vi "纳清蓝绿藻电极校准.vi"() -> ()   [LabVIEW 2016, in "斯坦道多参数.lvlib"]
uses:
  <vilib>/Utility/miscctls.llb/LVPointTypeDef.ctl
  <vilib>/Utility/miscctls.llb/LVPositionTypeDef.ctl
  <vilib>/Analysis/NI_AALBase.lvlib
panel:
  out "清扫间隔":u16
  out "清扫次数":u16
  in  "清扫模式":u16(ring) items=["自动清扫", "手动清扫", "启动一次清扫"]
  out "滤波设定":sgl
  in  "量程":u16(ring) items=["0-2000000", "0-200000"]
  out "第三点信号值":dbl
  out "第二点信号值":dbl
  out "第一点信号值":dbl
  out "报警信息":string
  out "通讯状态":string
  out "第三点校准值":dbl
  out "标液3":sgl
  out "第二点校准值":dbl
  out "第一点校准值":dbl
  in  "校准停止":bool
  in  "校准启动":bool
  in  "校准模式":u16(ring)=1 items=["两点校准", "单点校准", "三点校准"]
  out "最小值":sgl format="%#.2f"
  out "最大值":sgl format="%#.2f"
  out "波形图表":dbl(graph) caption="历史曲线"
  out "mean":dbl caption="均值" format="%#.2f"
  out "standard deviation":dbl caption="标准差" format="%#.2f"
  out "变异系数":dbl format="%#.6f"
  out "测量值":sgl format="%#.2f"
  out "提示":string
  out "标液2":sgl
  out "标液1":sgl
  out "原始光强数值":u16 caption="信号值"
  out "温度":dbl format="%#.2f"
  # "藻密度电极设定"
  # "℃"
  # "cells/mL"
  # "cells/mL"
  # "请选择校准模式:"
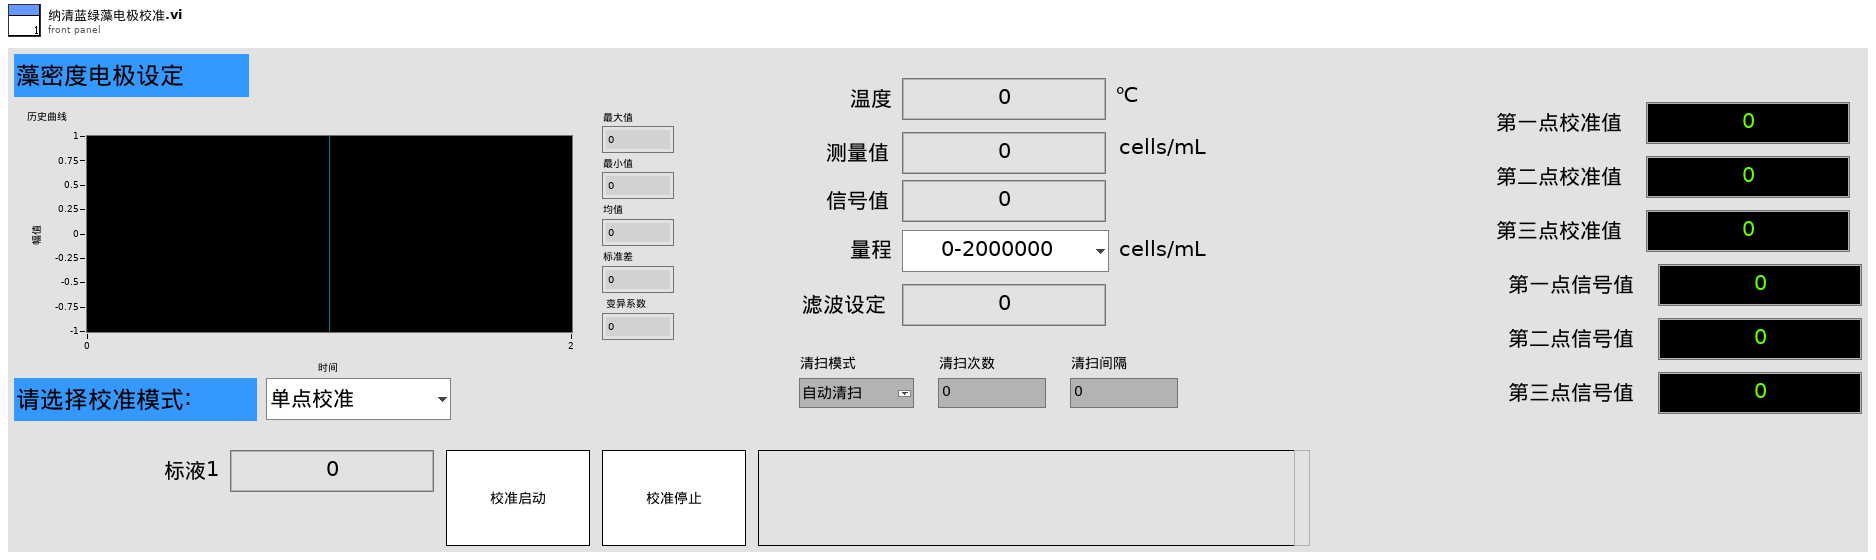
[diagram p1: front panel]
types:
  T1 = typedef "斯坦道多参数.lvlib/通知队列类型.ctl" = enum16{"pH", "DO", "DO2", "Cond", "Turb", "ORP", "叶绿素a", "藻密度", "COD"}
  T2 = typedef "LVPointTypeDef.ctl" = cluster{"Horizontal":i16, "Vertical":i16}
  T3 = cluster{"报警码":u16, "蓝绿藻":sgl, "温度数据":sgl, "原始光强数值":u16, "量程":u16, "平均次数":u16, "清扫模式":u16, "清扫次数":u16, "清扫间隔分钟":u16, "0X000B_NC":string, "产品名称":string, "序列号":string, "硬件版本":string, "软件版本":string, "通讯地址":u16, "波特率":u16, "设备类型":u16, "0X0026_NC":string, "校准量程":u16, "第一点原始光强":u16, "第一点校准数据":sgl, "第二点原始光强":u16, "第二点校准数据":sgl, "第三点原始光强":u16, "第三点校准数据":sgl, "探头校准命令":u16, "温度校准参数":sgl, "温度校准命令":u16}
  T4 = cluster{"pH":u32, "DO":u32, "Cond":u32, "Turb":u32, "叶绿素a":u32, "藻密度":u32, "ORP":u32, "COD":u32}
  T5 = typedef "LVPositionTypeDef.ctl" = cluster{"Left":i32, "Top":i32}
  T6 = enum8{"Enabled", "Disabled", "Disabled and Grayed Out"}
  T7 = cluster{"报警码":u16, "蓝绿藻":sgl, "温度数据":sgl, "原始光强数值":u16, "0X0006_NC":u16, "平均次数":u16, "清扫模式":u16, "清扫次数":u16, "清扫间隔分钟":u16, "0X000B_NC":string, "产品名称":string, "序列号":string, "硬件版本":string, "软件版本":string, "通讯地址":u16, "波特率":u16, "设备类型":u16, "0X0026_NC":string, "0X0030_NC":u16, "第一点原始光强":u16, "第一点校准数据":sgl, "第二点原始光强":u16, "第二点校准数据":sgl, "第三点原始光强":u16, "第三点校准数据":sgl, "探头校准命令":u16, "温度校准参数":sgl, "温度校准命令":u16}
  T8 = cluster{"ph":bool, "DO":bool, "Cond":bool, "Turb":bool, "叶绿素a":bool, "藻密度":bool, "ORP":bool, "COD":bool, "DO2":bool}
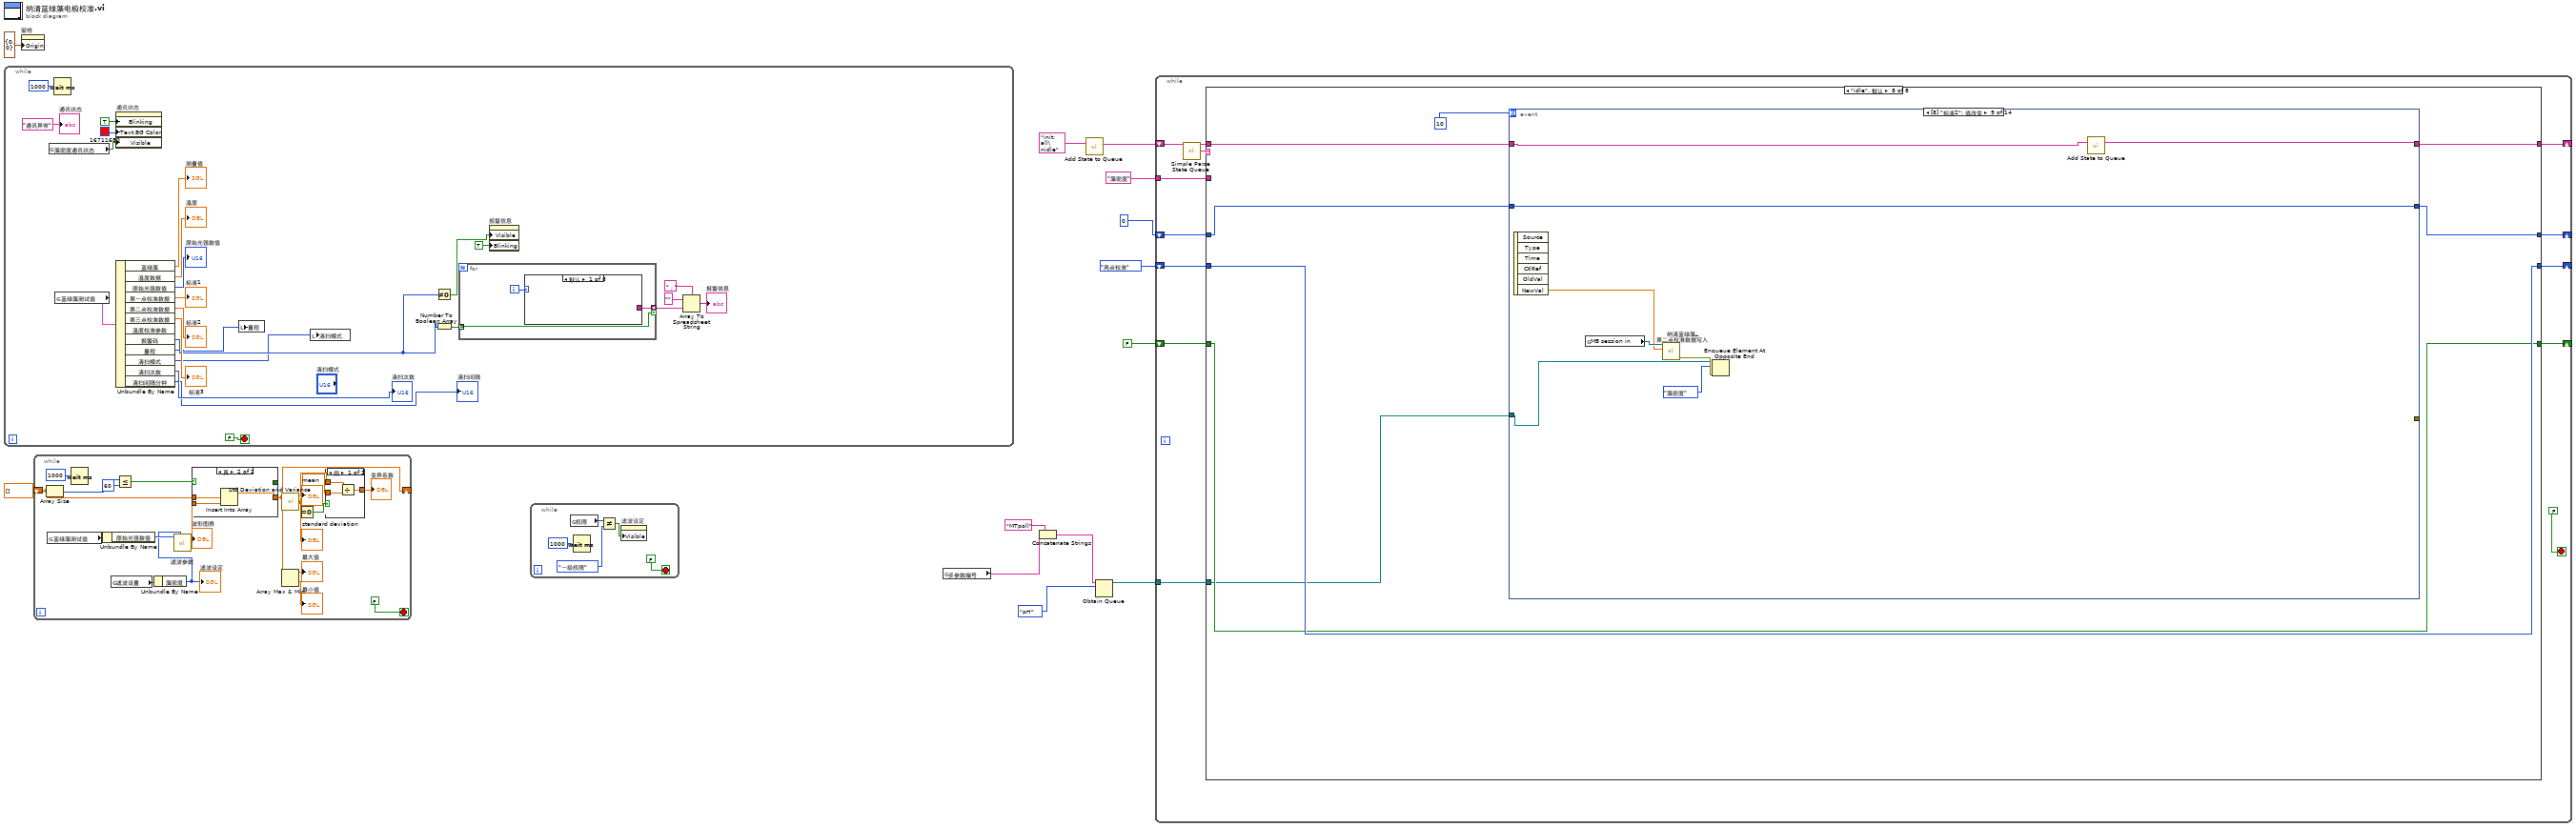
[diagram p0: block diagram]
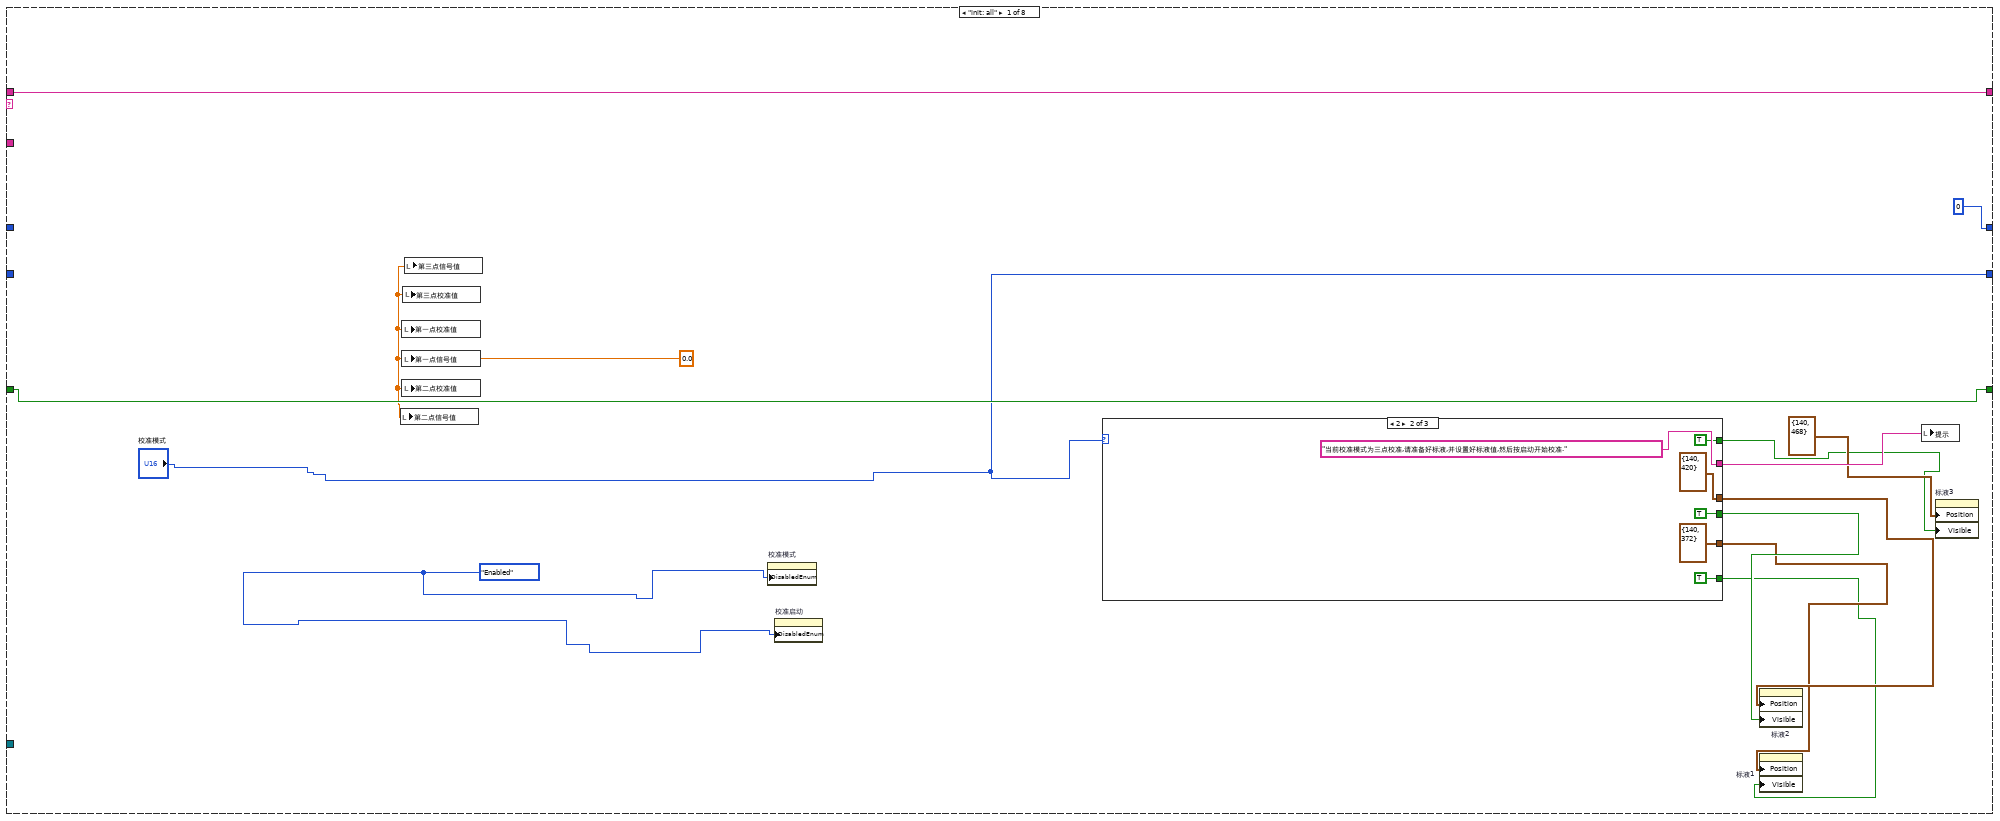
[diagram p2: hidden frame]
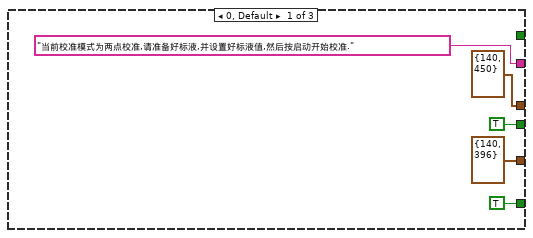
[diagram p3: hidden frame]
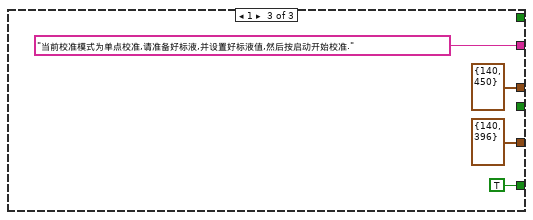
[diagram p4: hidden frame]
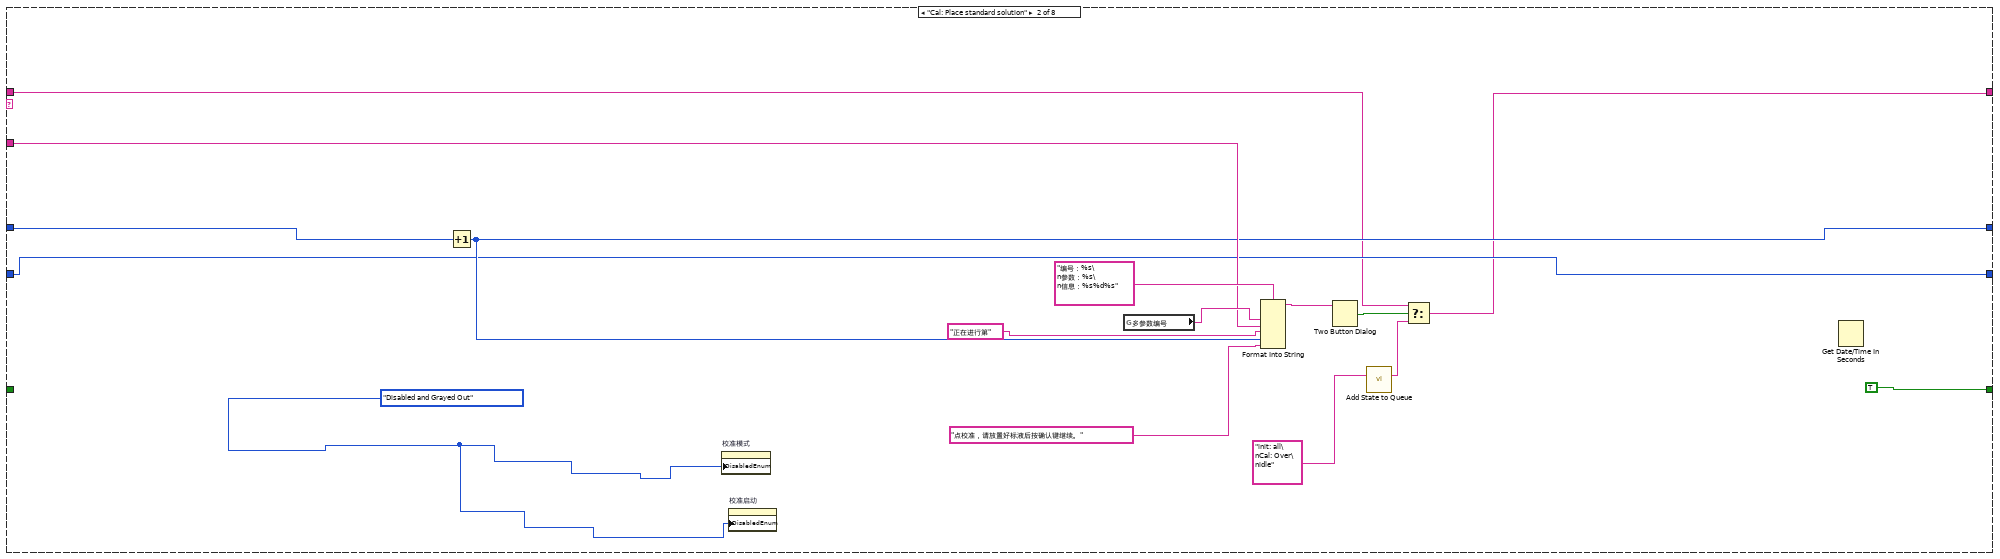
[diagram p5: hidden frame]
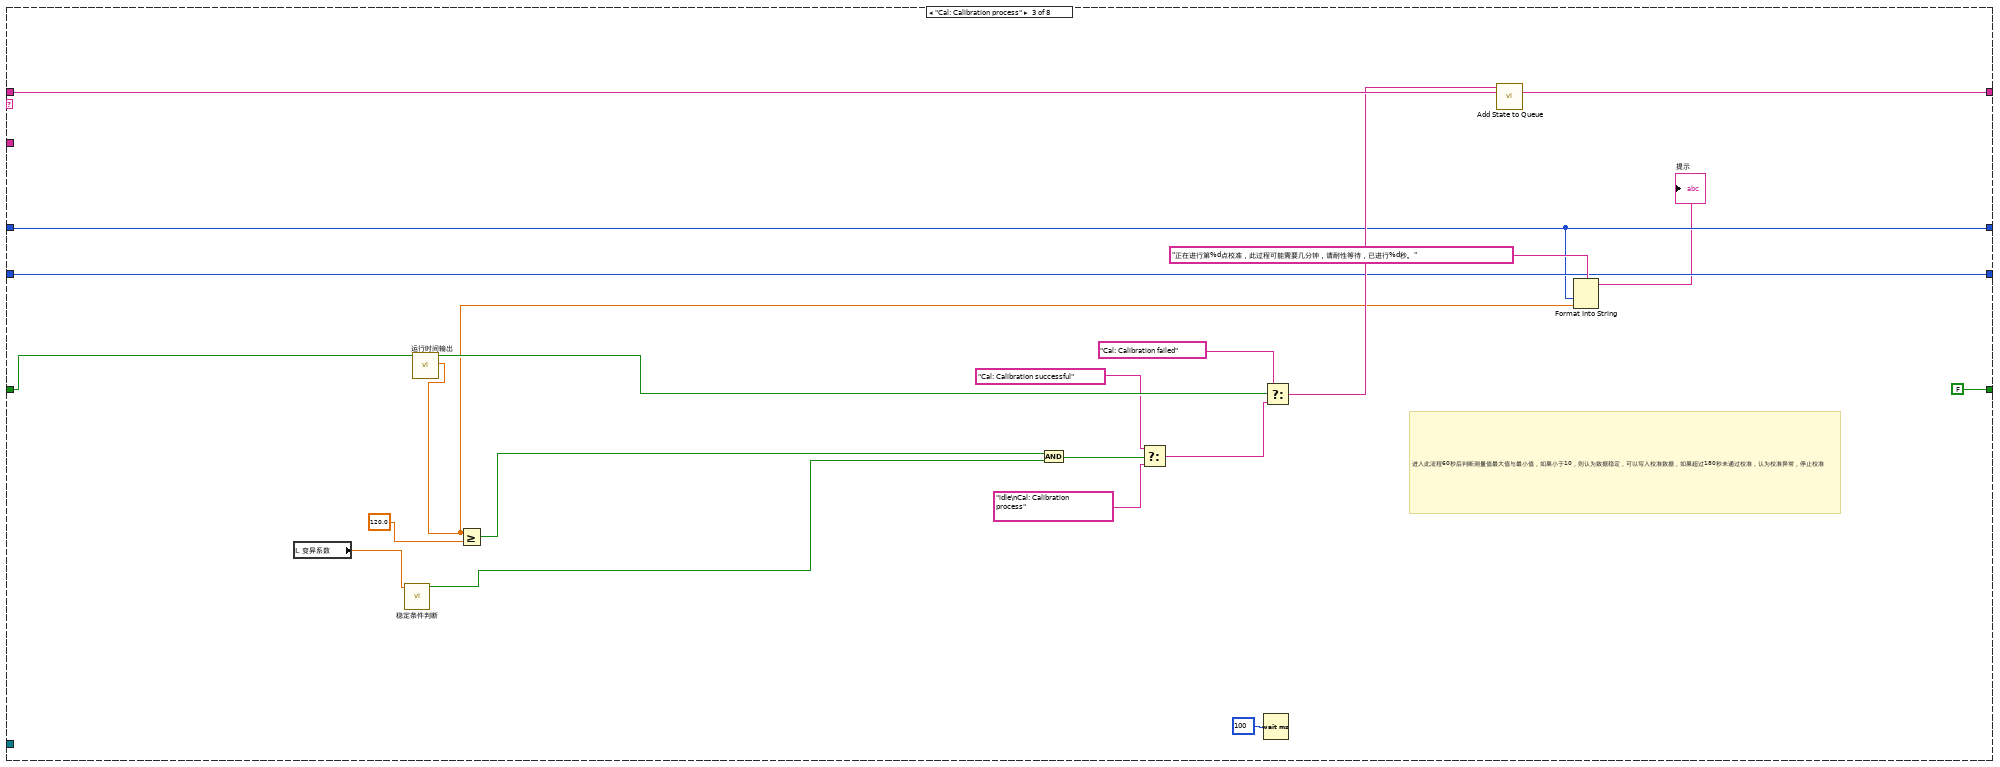
[diagram p6: hidden frame]
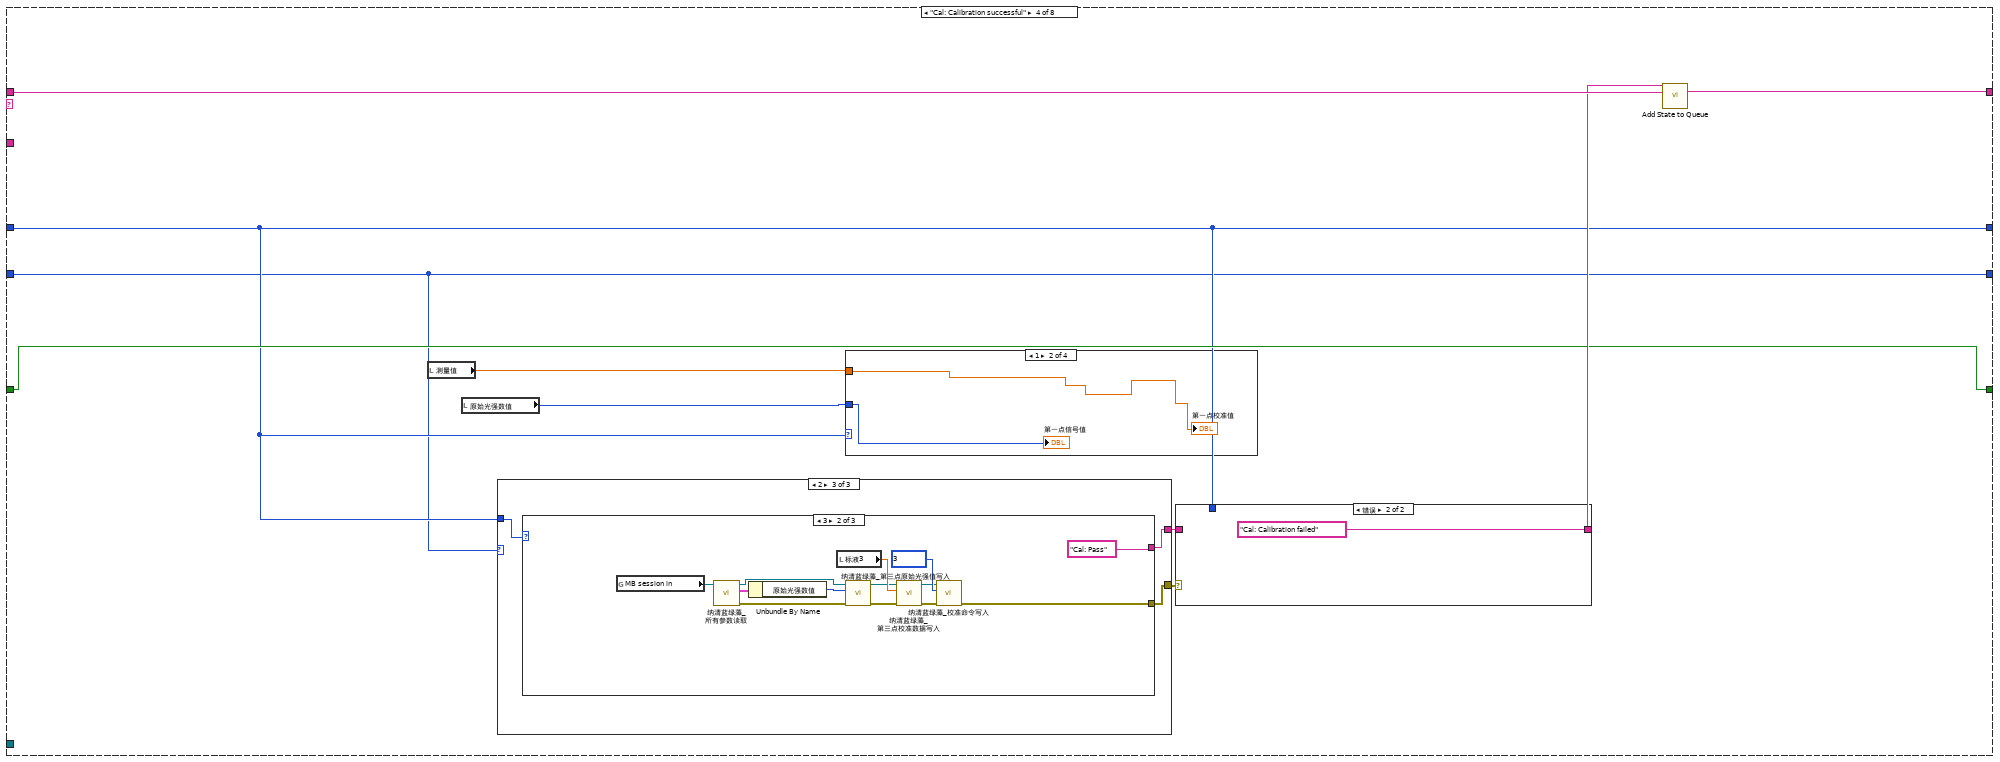
[diagram p7: hidden frame]
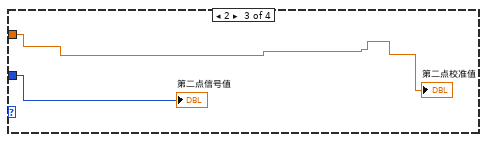
[diagram p9: hidden frame]
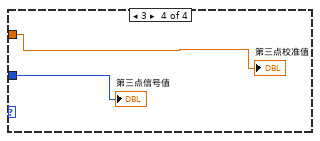
[diagram p10: hidden frame]
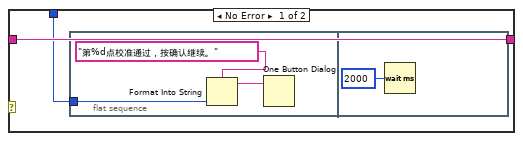
[diagram p11: hidden frame]
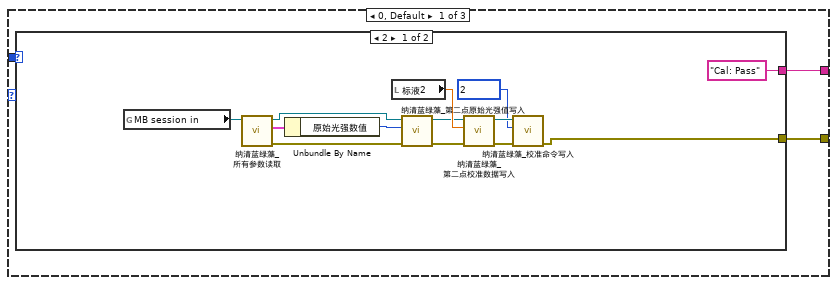
[diagram p12: hidden frame]
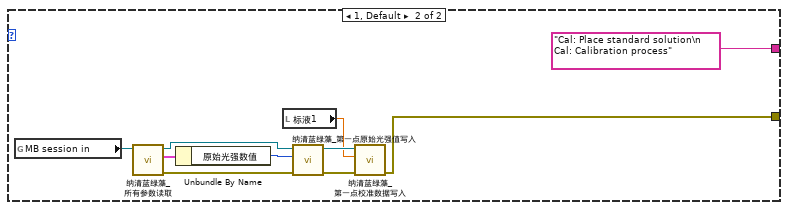
[diagram p13: hidden frame]
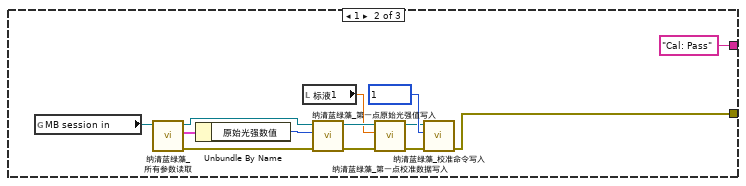
[diagram p14: hidden frame]
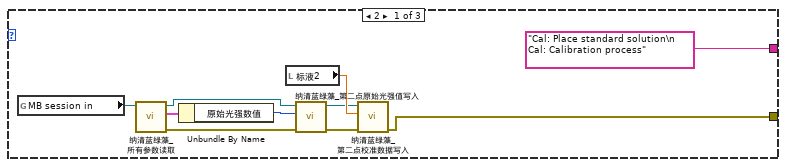
[diagram p15: hidden frame]
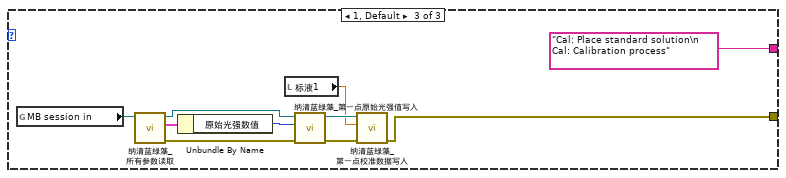
[diagram p16: hidden frame]
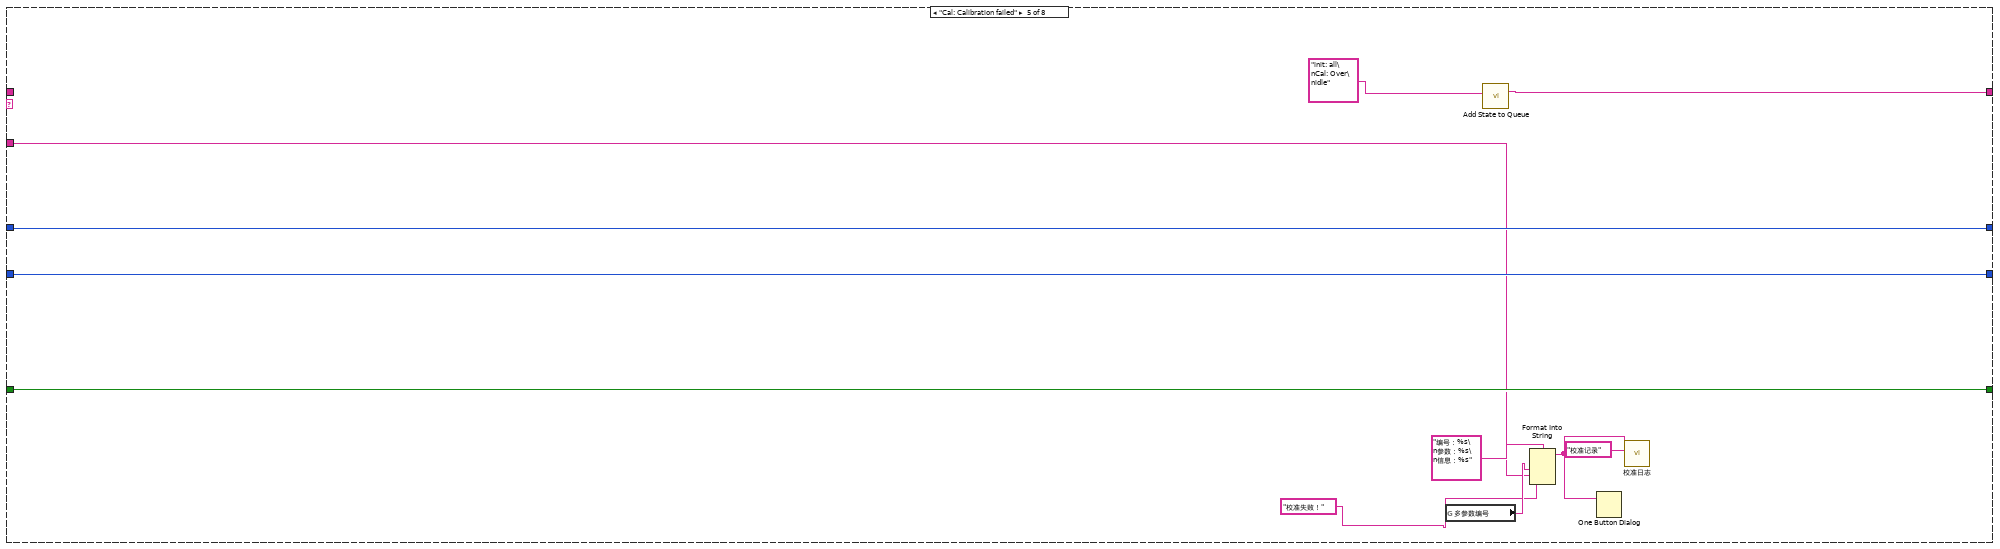
[diagram p17: hidden frame]
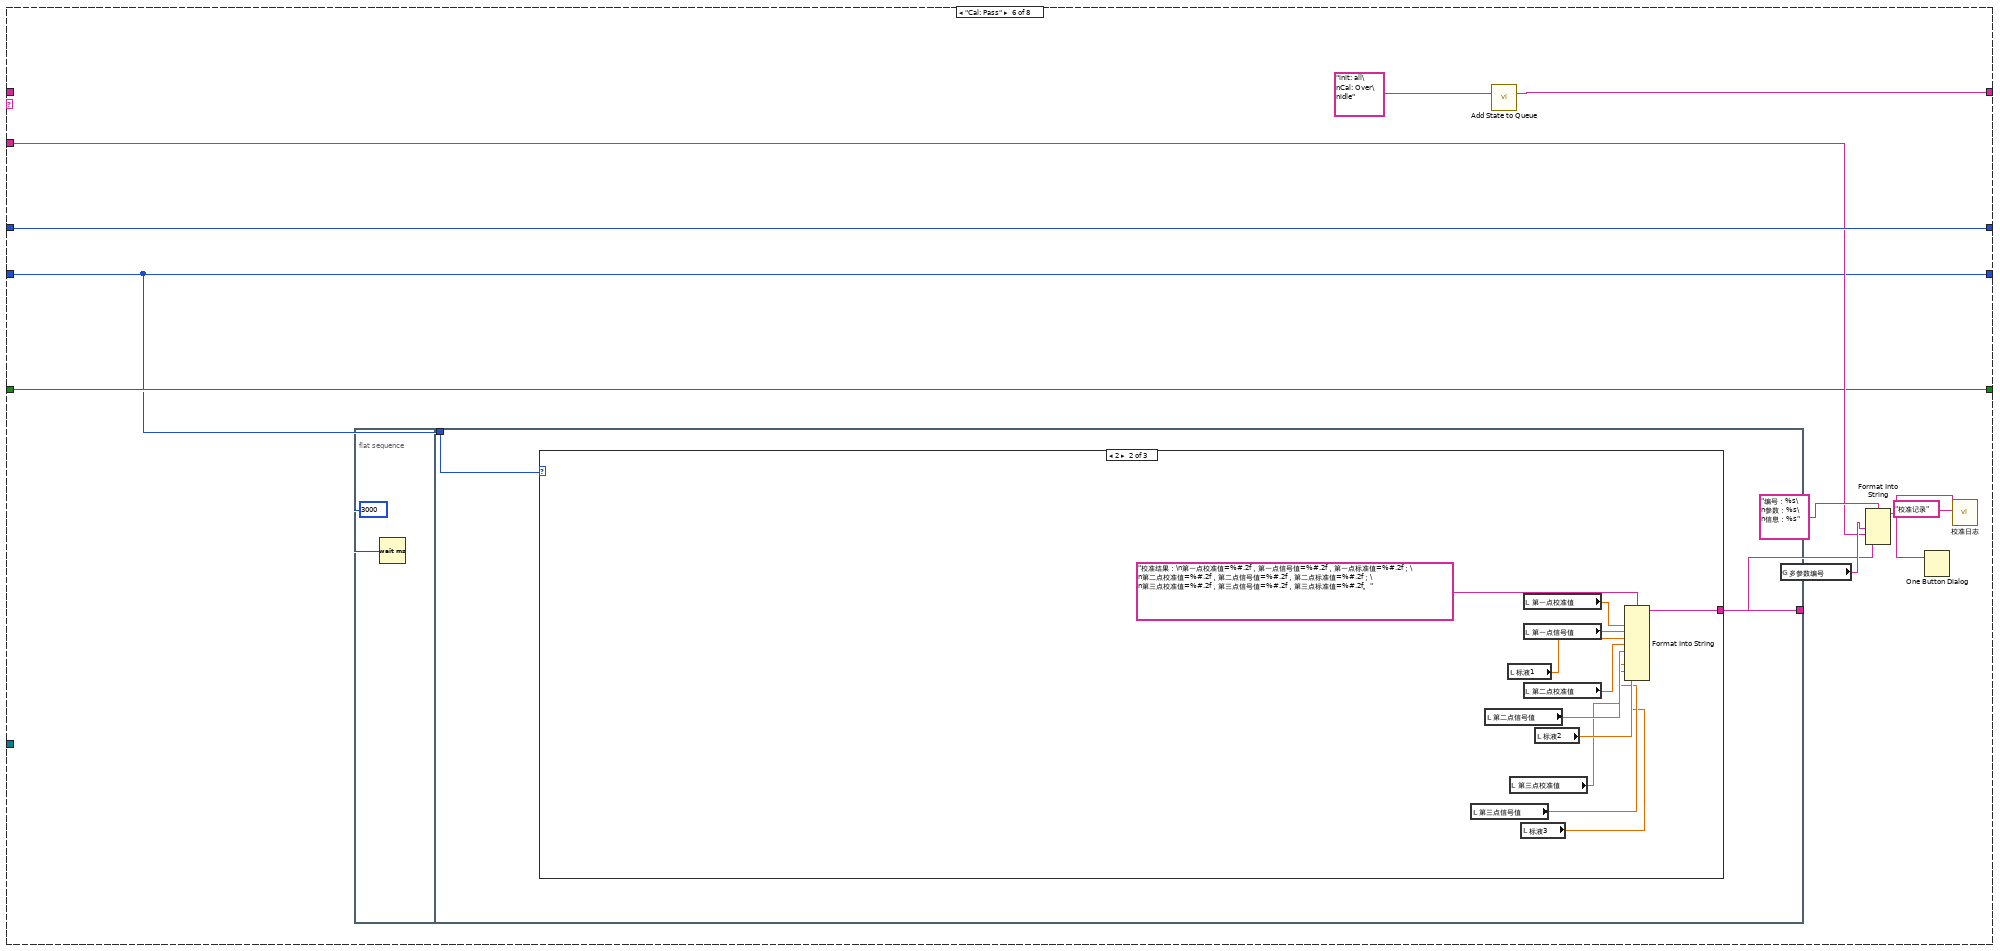
[diagram p18: hidden frame]
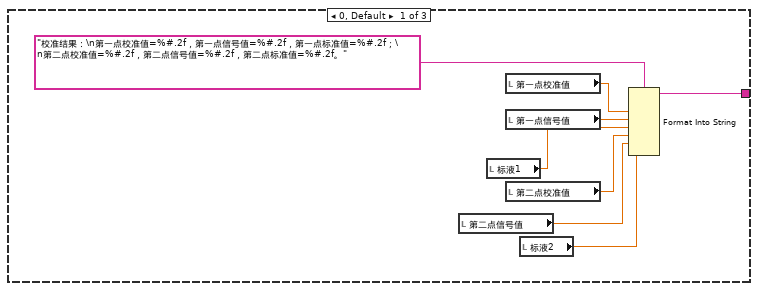
[diagram p19: hidden frame]
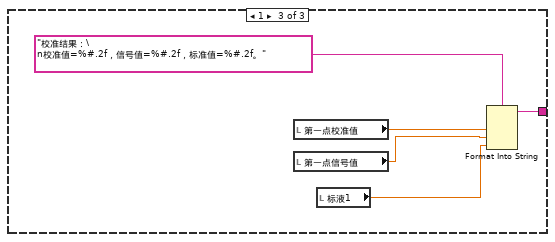
[diagram p20: hidden frame]
diagram:
  n1 = while {
    stop <- FALSE stop-if-true
    n2 = global read "多参数全局变量.vi" "藻密度通讯状态"() -> (w26:bool)
    n3 = Wait (ms)(milliseconds to wait=u32 1000 ("等待时间（毫秒）")) -> ()  [unwired: 1 out]
    n4 = global read "纳清过程全局变量.vi" "蓝绿藻测试值"() -> (w36:T3)
    n5 = property on="通讯状态" class="Str"("Blinking"=TRUE ("闪烁"), "Text.BG Color"=u32 16711680, "Visible"=w26) -> ()  [unwired: 2 in, 2 out]
    n6 = Unbundle By Name(w36) -> ("蓝绿藻"=→"测量值":sgl, "温度数据"=→"温度":sgl, "原始光强数值"=→"原始光强数值":u16, "第一点校准数据"=→"标液1":sgl, "第二点校准数据"=→"标液2":sgl, "第三点校准数据"=→"标液3":sgl, "报警码"=w18:u16, "量程"=w17:u16, "清扫模式"=w14:u16, "清扫次数"=→"清扫次数":u16, "清扫间隔分钟"=→"清扫间隔":u16)  [unwired: 1 out]
    n7 = local write "量程"(w17) -> ()
    n8 = local write "清扫模式"(w14) -> ()
    n9 = Not Equal To 0?(x=w18) -> (x != 0?=w20:bool)
    n10 = Number To Boolean Array(number=w18) -> (Boolean array=w25:bool[])
    n11 = for {
      tunnel: w25 -> [w39] mode=indexing
      tunnel: [w40] -> w24 mode=indexing if=w39
      i -> [w41]
      n12 = case shown="默认" w41 {
        tunnel: [_ "测量值超量程" "温度超量程" "光强信号超范围" "清扫中" "温度传感器故障" "电极故障" "内部电压基准故障"] -> w40
        frame Default {
        }
        frame 0 {
        }
        frame 2 {
        }
        frame 3 {
        }
        frame 4 {
        }
        frame 8 {
        }
        frame 9 {
        }
        frame 10 {
        }
      }
    }
    n13 = property on="报警信息" class="Str"("Visible"=w20, "Blinking"=TRUE ("闪烁")) -> ()  [unwired: 2 in, 2 out]
    n14 = Array To Spreadsheet String(delimiter (Tab)="；" ("分隔符(Tab)"), array=w24, 3:"" ("格式字符串")) -> (spreadsheet string=→"报警信息":string)
    "通讯状态" <- "通讯异常" ("当前串口")
  }
  n15 = property on="窗格" class="Pane"("Origin"=T2 {"Horizontal"=0, "Vertical"=0} ("原点")) -> ()  [unwired: 2 in, 2 out]
  n16 = while {
    shift-right: [w56] -> _
    shift-left: sgl[] [] -> [w62]
    stop <- FALSE stop-if-true
    n17 = Array Size(array=w62) -> (size(s)=w64:i32)
    n18 = global read "纳清过程全局变量.vi" "蓝绿藻测试值"() -> (w53:T3)
    n19 = Wait (ms)(milliseconds to wait=u32 1000 ("等待时间（毫秒）")) -> ()  [unwired: 1 out]
    n20 = Unbundle By Name(w53) -> ("原始光强数值"=w52:u16)
    n21 = global read "断电保存变量.vi" "滤波设置"() -> (w50:T4)
    n22 = Less Or Equal?(x=w64, y=60) -> (x <= y?=w63:bool)
    n23 = Unbundle By Name(w50) -> ("藻密度"=w49:u32)
    "滤波设定" <- w49
    n24 = call "滤波参数.vi"("滤波次数"=w49, "x"=w52) -> ("mode"=w51:dbl)  [unwired: 9 in]
    "波形图表" <- w51
    n25 = case shown="真" w63 {
      tunnel: w62 -> [w75 w78]
      tunnel: w51 -> [w73 w77]
      tunnel: [w71 w76] -> w56
      tunnel: [TRUE _] -> _
      frame False {
        n26 = Replace Array Subset(array=w75, new element=w73) -> (w74:sgl[])  [unwired: 1 in]
        n27 = Rotate 1D Array(1:w74, 2:-1 ("n")) -> (0:w71:sgl[])
      }
      frame True {
        n28 = Insert Into Array(array=w78, new element=w77) -> (w76:sgl[])  [unwired: 1 in]
      }
    }
    n29 = call <vilib>:"Std Deviation and Variance.vi"("X"=w56) -> ("mean"=w60:dbl, "standard deviation"=w59:dbl)  [unwired: 1 in, 1 out]
    "mean" <- w60
    "standard deviation" <- w59
    n30 = Array Max & Min(array=w56) -> (max value=→"最大值":sgl, min value=→"最小值":sgl)  [unwired: 2 out]
    n31 = Equal To 0?(x=w60) -> (x = 0?=w61:bool)
    n32 = case shown="假" w61 {
      tunnel: w59 -> [w69 _]
      tunnel: [w68 _] -> w58
      tunnel: w60 -> [w67 _]
      frame False {
        n33 = Divide(x=w69, y=w67) -> (x/y=w68:dbl)
      }
      frame True {
      }
    }
    "变异系数" <- w58
  }
  n34 = while {
    stop <- FALSE stop-if-true
    n35 = global read "多参数全局变量.vi" "权限"() -> (w82:enum16{"一级权限", "二级权限", "三级权限"})
    n36 = Wait (ms)(milliseconds to wait=u32 1000 ("等待时间（毫秒）")) -> ()  [unwired: 1 out]
    n37 = Not Equal?(x=w82, y=enum16{"一级权限", "二级权限", "三级权限"}."一级权限") -> (x != y?=w79:bool)
    n38 = property on="滤波设定" class="DigNum (严格)"("Visible"=w79) -> ()  [unwired: 2 in, 2 out]
  }
  n39 = global read "多参数全局变量.vi" "多参数编号"() -> (w3:string)
  n40 = Concatenate Strings("MTpoll" ("名称（未命名）"), w3) -> (w4:string)
  n41 = call "Add State to Queue.vi"("State(s) In (\"\")"="init: all\nidle" ("State(s) In (\"\")")) -> ("States Out"=w10:string)  [unwired: 14 in]
  n42 = Obtain Queue(name (unnamed)=w4, element data type=通知队列类型."pH" ("枚举")) -> (queue out=w2:refnum<queue>)  [unwired: 3 in, 2 out]
  n43 = while {
    shift-right: [w92] -> _
    shift-left: w10 -> [w96]
    shift-right: [w89] -> _
    shift-left: 0 -> [w91]
    tunnel: "藻密度" ("State(s) In (\"\")") -> [w90]
    shift-right: [w87] -> _
    shift-left: enum16{"两点校准", "单点校准", "三点校准"}."两点校准" ("校准模式") -> [w88]
    shift-right: [w85] -> _
    shift-left: FALSE -> [w86]
    tunnel: w2 -> [w84]
    stop <- FALSE stop-if-true
    n44 = call "Simple Parse State Queue.vi"("State Queue"=w96) -> ("Remain States"=w93:string, "Next State"=w94:string)  [unwired: 13 in]
    n45 = case shown="\"idle\", 默认" w94 {
      tunnel: w93 -> [w109 w128 w160 w169 _ _ w312 w323]
      tunnel: [w109 w127 w159 w168 w267 w272 w312 w322] -> w92
      tunnel: w91 -> [_ w136 w145 w163 w270 w281 w311 w320]
      tunnel: w90 -> [_ w137 _ _ w261 w277 _ _]
      tunnel: [0 w134 w145 w163 w270 w281 w311 w321] -> w89
      tunnel: w88 -> [_ w133 w146 w162 w269 w273 w310 w319]
      tunnel: ["校准模式" w133 w146 w162 w269 w273 w310 w319] -> w87
      tunnel: w86 -> [w107 _ w148 w164 w268 w276 w309 w317]
      tunnel: [w107 TRUE FALSE w164 w268 w276 w309 w317] -> w85
      tunnel: w84 -> [_ _ _ _ _ _ _ w316]
      frame "init: all" {
        w103 = T6."Enabled" ("禁用")
        w106 = 0.0 ("第一点校准值")
        n46 = local write "第二点信号值"(w106) -> ()
        n47 = local write "第一点校准值"(w106) -> ()
        n48 = local write "第一点信号值"(w106) -> ()
        n49 = local write "第二点校准值"(w106) -> ()
        n50 = local write "第三点校准值"(w106) -> ()
        n51 = local write "第三点信号值"(w106) -> ()
        n52 = property on="校准模式" class="Ring (严格)"("DisabledEnum"=w103) -> ()  [unwired: 2 in, 2 out]
        n53 = property on="校准启动" class="Bool"("DisabledEnum"=w103) -> ()  [unwired: 2 in, 2 out]
        n54 = case shown="2" "校准模式" {
          tunnel: ["当前校准模式为两点校准,请准备好标液,并设置好标液值,然后按启动开始校准." ("提示") "当前校准模式为三点校准,请准备好标液,并设置好标液值,然后按启动开始校准." ("提示") "当前校准模式为单点校准,请准备好标液,并设置好标液值,然后按启动开始校准." ("提示")] -> w105
          tunnel: [TRUE ("可见") TRUE ("可见") _] -> w99
          tunnel: [T5 {"Left"=140, "Top"=396} ("位置") T5 {"Left"=140, "Top"=372} ("位置") T5 {"Left"=140, "Top"=396} ("位置")] -> w98
          tunnel: [T5 {"Left"=140, "Top"=450} ("位置 2") T5 {"Left"=140, "Top"=420} ("位置 2") T5 {"Left"=140, "Top"=450} ("位置 2")] -> w100
          tunnel: [_ TRUE ("可见") _] -> w101
          tunnel: [TRUE ("可见") TRUE ("可见") TRUE ("可见")] -> w97
          frame 0, Default {
          }
          frame 2 {
          }
          frame 1 {
          }
        }
        n55 = property on="标液2" class="DigNum (严格)"("Position"=w100, "Visible"=w99) -> ()  [unwired: 2 in, 2 out]
        n56 = property on="标液1" class="DigNum (严格)"("Position"=w98, "Visible"=w97) -> ()  [unwired: 2 in, 2 out]
        n57 = local write "提示"(w105) -> ()
        n58 = property on="标液3" class="DigNum (严格)"("Position"=T5 {"Left"=140, "Top"=468} ("位置 3"), "Visible"=w101) -> ()  [unwired: 2 in, 2 out]
      }
      frame "Cal: Place standard solution" {
        w126 = T6."Disabled and Grayed Out" ("禁用")
        n59 = Increment(x=w136) -> (x+1=w134:i32)
        n60 = property on="校准模式" class="Ring (严格)"("DisabledEnum"=w126) -> ()  [unwired: 2 in, 2 out]
        n61 = property on="校准启动" class="Bool"("DisabledEnum"=w126) -> ()  [unwired: 2 in, 2 out]
        n62 = global read "多参数全局变量.vi" "多参数编号"() -> (w139:string)
        n63 = Format Into String(format string="编号：%s\n参数：%s\n信息：%s%d%s" ("格式字符串"), w139, w137, "正在进行第" ("消息"), w134, "点校准，请放置好标液后按确认键继续。" ("消息")) -> (resulting string=w131:string)  [unwired: 2 in, 1 out]
        n64 = Two Button Dialog(message=w131) -> (T button?=w130:bool)  [unwired: 2 in]
        n65 = call "Add State to Queue.vi"("State(s) In (\"\")"="init: all\nCal: Over\nidle" ("State(s) In (\"\")")) -> ("States Out"=w129:string)  [unwired: 14 in]
        n66 = Select(t=w128, s=w130, f=w129) -> (s? t:f=w127:string)
        n67 = Get Date/Time In Seconds() -> ()  [unwired: 1 out]
      }
      frame "Cal: Calibration process" {
        # "进入此流程60秒后判断测量值最大值与最小值，如果小于10，则认为数据稳定，可以写入校准数据，如果超过180秒未通过校准，认为校准异常，停止校准"
        n68 = local read "变异系数"() -> (w142:dbl)
        n69 = call "稳定条件判断.vi"("变异系数"=w142) -> ("布尔"=w141:bool)  [unwired: 10 in]
        n70 = call "运行时间输出.vi"("初始化"=w148) -> ("Elapsed Time (s)"=w144:dbl, "Time has Elapsed"=w161:bool)  [unwired: 9 in]
        n71 = Greater Or Equal?(x=w144, y=120.0) -> (x >= y?=w156:bool)
        n72 = And(x=w156, y=w141) -> (x .and. y?=w153:bool)
        n73 = Select(t="Cal: Calibration successful" ("State(s) In (\"\")"), s=w153, f="idle\nCal: Calibration process" ("State(s) In (\"\")")) -> (s? t:f=w152:string)
        n74 = Wait (ms)(milliseconds to wait=u32 100 ("等待时间（毫秒）")) -> ()  [unwired: 1 out]
        n75 = Select(t="Cal: Calibration failed" ("State(s) In (\"\")"), s=w161, f=w152) -> (s? t:f=w151:string)
        n76 = call "Add State to Queue.vi"("State(s) In Front (\"\")"=w151, "State(s) In (\"\")"=w160) -> ("States Out"=w159:string)  [unwired: 13 in]
        n77 = Format Into String(format string="正在进行第%d点校准，此过程可能需要几分钟，请耐性等待，已进行%d秒。" ("格式字符串"), w145, w144) -> (resulting string=→"提示":string)  [unwired: 2 in, 1 out]
      }
      frame "Cal: Calibration successful" {
        n78 = local read "测量值"() -> (w165:sgl)
        n79 = local read "原始光强数值"() -> (w166:u16)
        n80 = case shown="2" w162 {
          tunnel: [w187 w211 w224] -> w171
          tunnel: [w186 "Cal: Pass" ("State(s) In (\"\")") w225] -> w170
          tunnel: w163 -> [w185 _ w226]
          frame 0, Default {
            n81 = case shown="2" w185 {
              tunnel: [w188 w201] -> w187
              tunnel: ["Cal: Pass" ("State(s) In (\"\")") "Cal: Place standard solution\n Cal: Calibration process" ("State(s) In (\"\")")] -> w186
              frame 2 {
                n82 = global read "多参数全局变量.vi" "MB session in"() -> (w192:refnum<class "MB_Master.lvclass">)
                n83 = call "纳清蓝绿藻_所有参数读取.vi"("MB session in"=w192) -> ("error out"=w190:errorcluster, "输出值"=w193:T7, "MB session out"=w191:refnum<class "MB_Master.lvclass">)  [unwired: 8 in]
                n84 = Unbundle By Name(w193) -> ("原始光强数值"=w194:u16)
                n85 = local read "标液2"() -> (w199:sgl)
                n86 = call "纳清蓝绿藻_第二点原始光强值写入.vi"("error in (no error)"=w190, "数值"=w194, "MB session in"=w191) -> ("error out"=w195:errorcluster, "MB session out"=w196:refnum<class "MB_Master.lvclass">)  [unwired: 7 in]
                n87 = call "纳清蓝绿藻_第二点校准数据写入.vi"("error in (no error)"=w195, "数值"=w199, "MB session in"=w196) -> ("error out"=w197:errorcluster, "MB session out"=w198:refnum<class "MB_Master.lvclass">)  [unwired: 7 in]
                n88 = call "纳清蓝绿藻_校准命令写入.vi"("error in (no error)"=w197, "数值"=u16 2 ("starting address"), "MB session in"=w198) -> ("error out"=w188:errorcluster)  [unwired: 7 in, 1 out]
              }
              frame 1, Default {
                n89 = global read "多参数全局变量.vi" "MB session in"() -> (w207:refnum<class "MB_Master.lvclass">)
                n90 = call "纳清蓝绿藻_所有参数读取.vi"("MB session in"=w207) -> ("error out"=w209:errorcluster, "输出值"=w206:T7, "MB session out"=w208:refnum<class "MB_Master.lvclass">)  [unwired: 8 in]
                n91 = Unbundle By Name(w206) -> ("原始光强数值"=w205:u16)
                n92 = local read "标液1"() -> (w202:sgl)
                n93 = call "纳清蓝绿藻_第一点原始光强值写入.vi"("error in (no error)"=w209, "数值"=w205, "MB session in"=w208) -> ("error out"=w204:errorcluster, "MB session out"=w203:refnum<class "MB_Master.lvclass">)  [unwired: 7 in]
                n94 = call "纳清蓝绿藻_第一点校准数据写入.vi"("error in (no error)"=w204, "数值"=w202, "MB session in"=w203) -> ("error out"=w201:errorcluster)  [unwired: 7 in, 1 out]
              }
            }
          }
          frame 1 {
            n95 = global read "多参数全局变量.vi" "MB session in"() -> (w219:refnum<class "MB_Master.lvclass">)
            n96 = call "纳清蓝绿藻_所有参数读取.vi"("MB session in"=w219) -> ("error out"=w221:errorcluster, "输出值"=w218:T7, "MB session out"=w220:refnum<class "MB_Master.lvclass">)  [unwired: 8 in]
            n97 = Unbundle By Name(w218) -> ("原始光强数值"=w217:u16)
            n98 = local read "标液1"() -> (w212:sgl)
            n99 = call "纳清蓝绿藻_第一点原始光强值写入.vi"("error in (no error)"=w221, "数值"=w217, "MB session in"=w220) -> ("error out"=w216:errorcluster, "MB session out"=w215:refnum<class "MB_Master.lvclass">)  [unwired: 7 in]
            n100 = call "纳清蓝绿藻_第一点校准数据写入.vi"("error in (no error)"=w216, "数值"=w212, "MB session in"=w215) -> ("error out"=w214:errorcluster, "MB session out"=w213:refnum<class "MB_Master.lvclass">)  [unwired: 7 in]
            n101 = call "纳清蓝绿藻_校准命令写入.vi"("error in (no error)"=w214, "数值"=u16 1 ("starting address"), "MB session in"=w213) -> ("error out"=w211:errorcluster)  [unwired: 7 in, 1 out]
          }
          frame 2 {
            n102 = case shown="3" w226 {
              tunnel: [w227 w237 w250] -> w224
              tunnel: ["Cal: Place standard solution\n Cal: Calibration process" ("State(s) In (\"\")") "Cal: Pass" ("State(s) In (\"\")") "Cal: Place standard solution\n Cal: Calibration process" ("State(s) In (\"\")")] -> w225
              frame 2 {
                n103 = global read "多参数全局变量.vi" "MB session in"() -> (w230:refnum<class "MB_Master.lvclass">)
                n104 = call "纳清蓝绿藻_所有参数读取.vi"("MB session in"=w230) -> ("error out"=w228:errorcluster, "输出值"=w231:T7, "MB session out"=w229:refnum<class "MB_Master.lvclass">)  [unwired: 8 in]
                n105 = Unbundle By Name(w231) -> ("原始光强数值"=w232:u16)
                n106 = local read "标液2"() -> (w235:sgl)
                n107 = call "纳清蓝绿藻_第二点原始光强值写入.vi"("error in (no error)"=w228, "数值"=w232, "MB session in"=w229) -> ("error out"=w233:errorcluster, "MB session out"=w234:refnum<class "MB_Master.lvclass">)  [unwired: 7 in]
                n108 = call "纳清蓝绿藻_第二点校准数据写入.vi"("error in (no error)"=w233, "数值"=w235, "MB session in"=w234) -> ("error out"=w227:errorcluster)  [unwired: 7 in, 1 out]
              }
              frame 3 {
                n109 = global read "多参数全局变量.vi" "MB session in"() -> (w240:refnum<class "MB_Master.lvclass">)
                n110 = call "纳清蓝绿藻_所有参数读取.vi"("MB session in"=w240) -> ("error out"=w238:errorcluster, "输出值"=w241:T7, "MB session out"=w239:refnum<class "MB_Master.lvclass">)  [unwired: 8 in]
                n111 = Unbundle By Name(w241) -> ("原始光强数值"=w242:u16)
                n112 = local read "标液3"() -> (w248:sgl)
                n113 = call "纳清蓝绿藻_第三点原始光强值写入.vi"("error in (no error)"=w238, "数值"=w242, "MB session in"=w239) -> ("error out"=w243:errorcluster, "MB session out"=w244:refnum<class "MB_Master.lvclass">)  [unwired: 7 in]
                n114 = call "纳清蓝绿藻_第三点校准数据写入.vi"("error in (no error)"=w243, "数值"=w248, "MB session in"=w244) -> ("error out"=w245:errorcluster, "MB session out"=w246:refnum<class "MB_Master.lvclass">)  [unwired: 7 in]
                n115 = call "纳清蓝绿藻_校准命令写入.vi"("error in (no error)"=w245, "数值"=u16 3 ("starting address"), "MB session in"=w246) -> ("error out"=w237:errorcluster)  [unwired: 7 in, 1 out]
              }
              frame 1, Default {
                n116 = global read "多参数全局变量.vi" "MB session in"() -> (w256:refnum<class "MB_Master.lvclass">)
                n117 = call "纳清蓝绿藻_所有参数读取.vi"("MB session in"=w256) -> ("error out"=w258:errorcluster, "输出值"=w255:T7, "MB session out"=w257:refnum<class "MB_Master.lvclass">)  [unwired: 8 in]
                n118 = Unbundle By Name(w255) -> ("原始光强数值"=w254:u16)
                n119 = local read "标液1"() -> (w251:sgl)
                n120 = call "纳清蓝绿藻_第一点原始光强值写入.vi"("error in (no error)"=w258, "数值"=w254, "MB session in"=w257) -> ("error out"=w253:errorcluster, "MB session out"=w252:refnum<class "MB_Master.lvclass">)  [unwired: 7 in]
                n121 = call "纳清蓝绿藻_第一点校准数据写入.vi"("error in (no error)"=w253, "数值"=w251, "MB session in"=w252) -> ("error out"=w250:errorcluster)  [unwired: 7 in, 1 out]
              }
            }
          }
        }
        n122 = case shown="1" w163 {
          tunnel: w166 -> [_ w173 w175 w177]
          tunnel: w165 -> [_ w172 w174 w176]
          frame 0, Default {
          }
          frame 1 {
            "第一点信号值" <- w173
            "第一点校准值" <- w172
          }
          frame 2 {
            "第二点信号值" <- w175
            "第二点校准值" <- w174
          }
          frame 3 {
            "第三点信号值" <- w177
            "第三点校准值" <- w176
          }
        }
        n123 = case shown="错误" w171 {
          tunnel: w170 -> [w179 _]
          tunnel: [w179 "Cal: Calibration failed" ("State(s) In (\"\")")] -> w167
          tunnel: w163 -> [w178 _]
          frame No Error {
            n124 = flat-sequence {
              tunnel: w178 -> [w180]
              frame #0 {
                n125 = Format Into String(format string="第%d点校准通过，按确认继续。" ("格式字符串"), w180) -> (resulting string=w182:string)  [unwired: 2 in, 1 out]
                n126 = One Button Dialog(message=w182) -> ()  [unwired: 1 in, 1 out]
              }
              frame #1 {
                n127 = Wait (ms)(milliseconds to wait=u32 2000 ("等待时间（毫秒）")) -> ()  [unwired: 1 out]
              }
            }
          }
          frame Error {
          }
        }
        n128 = call "Add State to Queue.vi"("State(s) In Front (\"\")"=w167, "State(s) In (\"\")"=w169) -> ("States Out"=w168:string)  [unwired: 13 in]
      }
      frame "Cal: Calibration failed" {
        n129 = global read "多参数全局变量.vi" "多参数编号"() -> (w264:string)
        n130 = call "Add State to Queue.vi"("State(s) In (\"\")"="init: all\nCal: Over\nidle" ("State(s) In (\"\")")) -> ("States Out"=w267:string)  [unwired: 14 in]
        n131 = Format Into String(format string="编号：%s\n参数：%s\n信息：%s" ("格式字符串"), w264, w261, "校准失败！" ("消息")) -> (resulting string=w263:string)  [unwired: 2 in, 1 out]
        n132 = One Button Dialog(message=w263) -> ()  [unwired: 1 in, 1 out]
        n133 = call "校准日志.vi"("table"="校准记录", "日志信息"=w263) -> ()  [unwired: 9 in, 1 out]
      }
      frame "Cal: Pass" {
        n134 = flat-sequence {
          tunnel: [w284] -> w274
          tunnel: w273 -> [w283]
          frame #0 {
            n135 = Wait (ms)(milliseconds to wait=u32 3000 ("等待时间（毫秒）")) -> ()  [unwired: 1 out]
          }
          frame #1 {
            n136 = case shown="2" w283 {
              tunnel: [w292 w303 w308] -> w284
              frame 0, Default {
                n137 = local read "第二点信号值"() -> (w286:dbl)
                n138 = local read "标液1"() -> (w288:sgl)
                n139 = local read "第一点校准值"() -> (w290:dbl)
                n140 = local read "第一点信号值"() -> (w291:dbl)
                n141 = local read "第二点校准值"() -> (w287:dbl)
                n142 = local read "标液2"() -> (w285:sgl)
                n143 = Format Into String(format string="校准结果：\n第一点校准值=%#.2f，第一点信号值=%#.2f，第一点标准值=%#.2f；\n第二点校准值=%#.2f，第二点信号值=%#.2f，第二点标准值=%#.2f。" ("提示"), w290, w291, w288, w287, w286, w285) -> (resulting string=w292:string)  [unwired: 2 in, 1 out]
              }
              frame 2 {
                n144 = local read "第三点信号值"() -> (w294:dbl)
                n145 = local read "第二点信号值"() -> (w297:dbl)
                n146 = local read "标液1"() -> (w299:sgl)
                n147 = local read "第三点校准值"() -> (w295:dbl)
                n148 = local read "标液3"() -> (w293:sgl)
                n149 = local read "第一点校准值"() -> (w301:dbl)
                n150 = local read "第一点信号值"() -> (w302:dbl)
                n151 = local read "第二点校准值"() -> (w298:dbl)
                n152 = local read "标液2"() -> (w296:sgl)
                n153 = Format Into String(format string="校准结果：\n第一点校准值=%#.2f，第一点信号值=%#.2f，第一点标准值=%#.2f；\n第二点校准值=%#.2f，第二点信号值=%#.2f，第二点标准值=%#.2f；\n第三点校准值=%#.2f，第三点信号值=%#.2f，第三点标准值=%#.2f。" ("提示"), w301, w302, w299, w298, w297, w296, w295, w294, w293) -> (resulting string=w303:string)  [unwired: 2 in, 1 out]
              }
              frame 1 {
                n154 = local read "第一点校准值"() -> (w307:dbl)
                n155 = local read "第一点信号值"() -> (w305:dbl)
                n156 = local read "标液1"() -> (w304:sgl)
                n157 = Format Into String(format string="校准结果：\n校准值=%#.2f，信号值=%#.2f，标准值=%#.2f。" ("提示"), w307, w305, w304) -> (resulting string=w308:string)  [unwired: 2 in, 1 out]
              }
            }
          }
        }
        n158 = call "Add State to Queue.vi"("State(s) In (\"\")"="init: all\nCal: Over\nidle" ("State(s) In (\"\")")) -> ("States Out"=w272:string)  [unwired: 14 in]
        n159 = global read "多参数全局变量.vi" "多参数编号"() -> (w278:string)
        n160 = Format Into String(format string="编号：%s\n参数：%s\n信息：%s" ("格式字符串"), w278, w277, w274) -> (resulting string=w275:string)  [unwired: 2 in, 1 out]
        n161 = One Button Dialog(message=w275) -> ()  [unwired: 1 in, 1 out]
        n162 = call "校准日志.vi"("table"="校准记录", "日志信息"=w275) -> ()  [unwired: 9 in, 1 out]
      }
      frame "Cal: Over" {
        n163 = global read "多参数全局变量.vi" "校准运行状态"() -> (w314:T8)
        n164 = Bundle By Name(cluster=w314, "藻密度"=FALSE ("Cond")) -> (w315:T8)
        n165 = global write "多参数全局变量.vi" "校准运行状态"(w315) -> ()
      }
      frame "idle", Default {
        n166 = event shown="[8] \"标液2\": 值改变" {
          selector: _ -> [_ _ _ _ _ _ _ _ _ _ _ _ _ _]
          dyn-events: _ -> [_ _ _ _ _ _ _ _ _ _ _ _ _ _]
          timeout: 10 -> [_ _ _ _ _ _ _ _ _ _ _ _ _ _]
          tunnel: w323 -> [w326 w330 w335 w342 w348 w356 w364 w372 w380 w388 w393 w404 w414 _]
          tunnel: [w325 w329 w336 w343 w352 w360 w368 w376 w384 w392 w395 w406 w413 w419] -> w322
          tunnel: [w324 w327 w337 w344 w351 w359 w367 w375 w383 w391 w394 w405 w411 w420] -> w321
          tunnel: w320 -> [w324 w327 w337 w344 w351 w359 w367 w375 w383 w391 w394 w405 w411 w420]
          tunnel: [_ _ _ _ _ _ _ _ _ _ _ _ w407 _] -> _
          tunnel: w316 -> [_ _ _ _ w346 w354 w362 w370 w378 w386 _ w400 _ _]
          event Timeout {
            n167 = event-data() -> ()  [unwired: 1 in, 3 out]
            n168 = call "Add State to Queue.vi"("State(s) In (\"\")"=w326) -> ("States Out"=w325:string)  [unwired: 14 in]
          }
          event "校准模式": Value Change {
            n169 = event-data() -> ()  [unwired: 1 in, 6 out]
            n170 = call "Add State to Queue.vi"("State(s) In (\"\")"=w330, "State(s) At Back (\"\")"="init: all\nidle" ("State(s) In (\"\")")) -> ("States Out"=w329:string)  [unwired: 13 in]
          }
          event "标液1", "标液2", "标液3", "滤波设定": Mouse Down {
            n171 = event-data() -> ("CtlRef"=w334:refnum<vi>)  [unwired: 1 in, 7 out]
            n172 = property class="DigNum (严格)"(reference=w334) -> (reference out=w331:refnum<vi>, "Value"=w332:sgl)  [unwired: 1 in, 1 out]
            n173 = call "数字键盘.vi"("OldNumber"=w332) -> ("NewNumber"=w333:dbl)  [unwired: 1 in]
            n174 = property class="DigNum (严格)"(reference=w331, "Val(Sgnl)"=w333) -> ()  [unwired: 1 in, 2 out]
            n175 = call "Add State to Queue.vi"("State(s) In (\"\")"=w335) -> ("States Out"=w336:string)  [unwired: 14 in]
          }
          event "清扫次数", "清扫间隔": Mouse Down {
            n176 = event-data() -> ("CtlRef"=w341:refnum<vi>)  [unwired: 1 in, 7 out]
            n177 = property class="DigNum (严格)"(reference=w341) -> (reference out=w338:refnum<vi>, "Value"=w339:u16)  [unwired: 1 in, 1 out]
            n178 = call "数字键盘.vi"("OldNumber"=w339) -> ("NewNumber"=w340:dbl)  [unwired: 1 in]
            n179 = property class="DigNum (严格)"(reference=w338, "Val(Sgnl)"=w340) -> ()  [unwired: 1 in, 2 out]
            n180 = call "Add State to Queue.vi"("State(s) In (\"\")"=w342) -> ("States Out"=w343:string)  [unwired: 14 in]
          }
          event "标液1": Value Change {
            n181 = event-data() -> ("NewVal"=w349:sgl)  [unwired: 1 in, 5 out]
            n182 = global read "多参数全局变量.vi" "MB session in"() -> (w350:refnum<class "MB_Master.lvclass">)
            n183 = call "纳清蓝绿藻_第一点校准数据写入.vi"("数值"=w349, "MB session in"=w350) -> ("error out"=w347:errorcluster)  [unwired: 8 in, 1 out]
            n184 = Enqueue Element At Opposite End(queue=w346, element=通知队列类型."藻密度" ("枚举"), error in (no error)=w347) -> ()  [unwired: 1 in, 3 out]
            n185 = call "Add State to Queue.vi"("State(s) In (\"\")"=w348) -> ("States Out"=w352:string)  [unwired: 14 in]
          }
          event "清扫模式": Value Change {
            n186 = event-data() -> ("NewVal"=w357:u16)  [unwired: 1 in, 5 out]
            n187 = global read "多参数全局变量.vi" "MB session in"() -> (w358:refnum<class "MB_Master.lvclass">)
            n188 = call "纳清蓝绿藻_清扫模式写入.vi"("清扫模式"=w357, "MB session in"=w358) -> ("error out"=w355:errorcluster)  [unwired: 8 in, 1 out]
            n189 = Enqueue Element At Opposite End(queue=w354, element=通知队列类型."藻密度" ("枚举"), error in (no error)=w355) -> ()  [unwired: 1 in, 3 out]
            n190 = call "Add State to Queue.vi"("State(s) In (\"\")"=w356) -> ("States Out"=w360:string)  [unwired: 14 in]
          }
          event "清扫次数": Value Change {
            n191 = event-data() -> ("NewVal"=w365:u16)  [unwired: 1 in, 5 out]
            n192 = global read "多参数全局变量.vi" "MB session in"() -> (w366:refnum<class "MB_Master.lvclass">)
            n193 = call "纳清蓝绿藻_清扫次数写入.vi"("数值"=w365, "MB session in"=w366) -> ("error out"=w363:errorcluster)  [unwired: 8 in, 1 out]
            n194 = Enqueue Element At Opposite End(queue=w362, element=通知队列类型."叶绿素a" ("枚举"), error in (no error)=w363) -> ()  [unwired: 1 in, 3 out]
            n195 = call "Add State to Queue.vi"("State(s) In (\"\")"=w364) -> ("States Out"=w368:string)  [unwired: 14 in]
          }
          event "清扫间隔": Value Change {
            n196 = event-data() -> ("NewVal"=w373:u16)  [unwired: 1 in, 5 out]
            n197 = global read "多参数全局变量.vi" "MB session in"() -> (w374:refnum<class "MB_Master.lvclass">)
            n198 = call "纳清蓝绿藻_清扫间隔写入.vi"("数值"=w373, "MB session in"=w374) -> ("error out"=w371:errorcluster)  [unwired: 8 in, 1 out]
            n199 = Enqueue Element At Opposite End(queue=w370, element=通知队列类型."藻密度" ("枚举"), error in (no error)=w371) -> ()  [unwired: 1 in, 3 out]
            n200 = call "Add State to Queue.vi"("State(s) In (\"\")"=w372) -> ("States Out"=w376:string)  [unwired: 14 in]
          }
          event "标液2": Value Change {
            n201 = event-data() -> ("NewVal"=w381:sgl)  [unwired: 1 in, 5 out]
            n202 = global read "多参数全局变量.vi" "MB session in"() -> (w382:refnum<class "MB_Master.lvclass">)
            n203 = call "纳清蓝绿藻_第二点校准数据写入.vi"("数值"=w381, "MB session in"=w382) -> ("error out"=w379:errorcluster)  [unwired: 8 in, 1 out]
            n204 = Enqueue Element At Opposite End(queue=w378, element=通知队列类型."藻密度" ("枚举"), error in (no error)=w379) -> ()  [unwired: 1 in, 3 out]
            n205 = call "Add State to Queue.vi"("State(s) In (\"\")"=w380) -> ("States Out"=w384:string)  [unwired: 14 in]
          }
          event "标液3": Value Change {
            n206 = event-data() -> ("NewVal"=w389:sgl)  [unwired: 1 in, 5 out]
            n207 = global read "多参数全局变量.vi" "MB session in"() -> (w390:refnum<class "MB_Master.lvclass">)
            n208 = call "纳清蓝绿藻_第三点校准数据写入.vi"("数值"=w389, "MB session in"=w390) -> ("error out"=w387:errorcluster)  [unwired: 8 in, 1 out]
            n209 = Enqueue Element At Opposite End(queue=w386, element=通知队列类型."藻密度" ("枚举"), error in (no error)=w387) -> ()  [unwired: 1 in, 3 out]
            n210 = call "Add State to Queue.vi"("State(s) In (\"\")"=w388) -> ("States Out"=w392:string)  [unwired: 14 in]
          }
          event "滤波设定": Value Change {
            n211 = event-data() -> ()  [unwired: 1 in, 6 out]
            n212 = flat-sequence {
              frame #0 {
                n213 = global read "断电保存变量.vi" "滤波设置"() -> (w398:T4)
                n214 = local read "滤波设定"() -> (w396:sgl)
                n215 = Bundle By Name(cluster=w398, "藻密度"=w396) -> (w397:T4)
                n216 = global write "断电保存变量.vi" "滤波设置"(w397) -> ()
              }
              frame #1 {
                n217 = call "配置文件保存.vi"() -> ()  [unwired: 12 in]
              }
            }
            n218 = call "Add State to Queue.vi"("State(s) In (\"\")"=w393) -> ("States Out"=w395:string)  [unwired: 14 in]
          }
          event "量程": Value Change {
            n219 = event-data() -> ("NewVal"=w402:u16)  [unwired: 1 in, 5 out]
            n220 = global read "多参数全局变量.vi" "MB session in"() -> (w403:refnum<class "MB_Master.lvclass">)
            n221 = call "纳清蓝绿藻_量程写入.vi"("数值"=w402, "MB session in"=w403) -> ("error out"=w401:errorcluster)  [unwired: 8 in, 1 out]
            n222 = Enqueue Element At Opposite End(queue=w400, element=通知队列类型."藻密度" ("枚举"), error in (no error)=w401) -> ()  [unwired: 1 in, 3 out]
            n223 = call "Add State to Queue.vi"("State(s) In (\"\")"=w404) -> ("States Out"=w406:string)  [unwired: 14 in]
          }
          event "校准启动": Value Change {
            n224 = event-data() -> ()  [unwired: 1 in, 6 out]
            n225 = global read "纳清过程全局变量.vi" "蓝绿藻测试值"() -> (w409:T3)
            n226 = Unbundle By Name(w409) -> ("量程"=w408:u16)
            n227 = global read "多参数全局变量.vi" "MB session in"() -> (w410:refnum<class "MB_Master.lvclass">)
            n228 = call "纳清蓝绿藻_校准量程写入.vi"("数值"=w408, "MB session in"=w410) -> ("error out"=w407:errorcluster)  [unwired: 8 in, 1 out]
            n229 = call "Add State to Queue.vi"("State(s) In (\"\")"=w414, "State(s) At Back (\"\")"="init: all\nCal: Place standard solution\n Cal: Calibration process\nidle" ("State(s) In (\"\")")) -> ("States Out"=w413:string)  [unwired: 13 in]
          }
          event "校准停止": Value Change {
            n230 = event-data() -> ()  [unwired: 1 in, 6 out]
            n231 = global read "多参数全局变量.vi" "校准运行状态"() -> (w416:T8)
            n232 = Bundle By Name(cluster=w416, "藻密度"=TRUE ("Cond")) -> (w417:T8)
            n233 = global write "多参数全局变量.vi" "校准运行状态"(w417) -> ()
            n234 = call "Add State to Queue.vi"("State(s) In (\"\")"="init: all\nCal: Over\nidle" ("State(s) In (\"\")")) -> ("States Out"=w419:string)  [unwired: 14 in]
          }
        }
      }
    }
  }
